vi "CAN_MotorControl.vi"(5 "sbCANopenBaseClass in":refnum<class "sbCANopenBaseClass.lvclass">, 6 "Current":i32=10, 7 "error in (no error)":errorcluster) -> (0 "CANopen Session Out":refnum<class "sbCANopenBaseClass.lvclass">, 1 "Status":T2, 2 "Data Output":T1, 3 "Actual Velocity":i32, 4 "error out":errorcluster)   [LabVIEW 2017]
uses:
  <vilib>/addons/Maxon Motor/EPOS2 CANopen/CANopen/sbCANopenBaseClass.lvclass
  <vilib>/addons/Maxon Motor/EPOS2 CANopen/EPOS2 Support Files/Typedefs/EPOS2 Status Word PVM.ctl
  <vilib>/addons/Maxon Motor/EPOS2 CANopen/EPOS2 Support Files/Typedefs/EPOS2 Data Output Current.ctl
  <vilib>/addons/Maxon Motor/EPOS2 CANopen/EPOS2 Support Files/Typedefs/EPOS2 Control Word PVM.ctl
  <vilib>/addons/Maxon Motor/EPOS2 CANopen/EPOS2 Support Files/Polymorphic SubVIs/Write PDO/EPOS2 Current Mode Write.vi
  <vilib>/addons/Maxon Motor/EPOS2 CANopen/EPOS2 Support Files/Polymorphic SubVIs/Read PDO/EPOS2 Current Mode Read.vi
  <vilib>/addons/Maxon Motor/EPOS2 CANopen/EPOS2 Library.lvlib
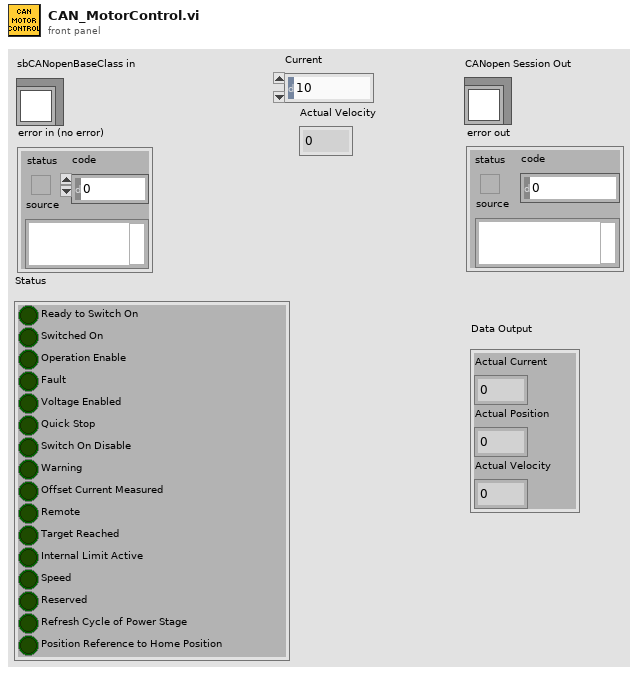
[diagram p1: front panel]
types:
  T1 = typedef "EPOS2 Library.lvlib/EPOS2 Data Output Current.ctl" = cluster{"Actual Current":i16, "Actual Position":i32, "Actual Velocity":i32}
  T2 = typedef "EPOS2 Library.lvlib/EPOS2 Status Word PVM.ctl" = cluster{"Ready to Switch On":bool, "Switched On":bool, "Operation Enable":bool, "Fault":bool, "Voltage Enabled":bool, "Quick Stop":bool, "Switch On Disable":bool, "Warning":bool, "Offset Current Measured":bool, "Remote":bool, "Target Reached":bool, "Internal Limit Active":bool, "Speed":bool, "Reserved":bool, "Refresh Cycle of Power Stage":bool, "Position Reference to Home Position":bool}
  T3 = typedef "EPOS2 Library.lvlib/EPOS2 Control Word PVM.ctl" = cluster{"Switch On":bool, "Enable Voltage":bool, "Quick Stop":bool, "Enable Operation":bool, "Reserved 0":bool, "Reserved 1":bool, "Reserved 2":bool, "Fault Reset":bool, "Halt":bool}
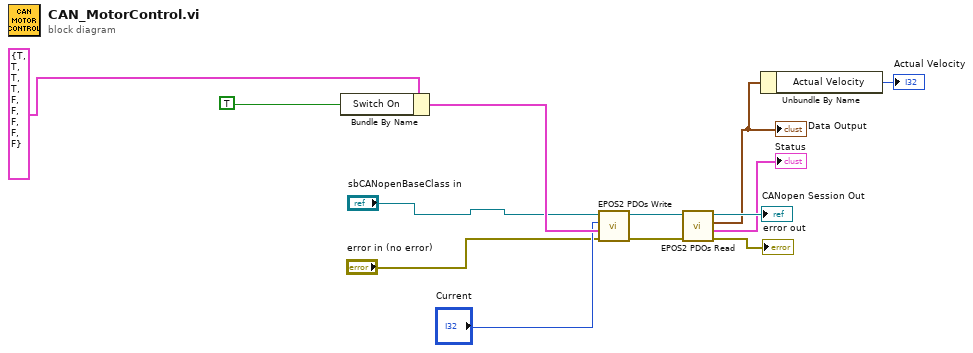
[diagram p0: block diagram]
diagram:
  n1 = Bundle By Name(cluster=T3 {"Switch On"=TRUE, "Enable Voltage"=TRUE, "Quick Stop"=TRUE, "Enable Operation"=TRUE, "Reserved 0"=FALSE, "Reserved 1"=FALSE, "Reserved 2"=FALSE, "Fault Reset"=FALSE, "Halt"=FALSE} ("Control Word"), "Switch On"=TRUE) -> (w12:T3)
  n2 = call-poly <vilib>:"EPOS2 PDOs Write.vi"("error in"="error in (no error)", "Control Word"=w12, "Current"="Current", "CANopen Session In"="sbCANopenBaseClass in") -> ("error out"=w9:errorcluster, "CANopen Session Out"=w11:refnum<class "sbCANopenBaseClass.lvclass">)  [unwired: 6 in]
  n3 = call-poly <vilib>:"EPOS2 PDOs Read.vi"("error in"=w9, "CANopen Session In"=w11) -> ("error out"=→"error out":errorcluster, "Statusword"=→"Status":T2, "Data Output"=w4:T1, "CANopen Session Out"=→"CANopen Session Out":refnum<class "sbCANopenBaseClass.lvclass">)  [unwired: 6 in]
  "Data Output" <- w4
  n4 = Unbundle By Name(w4) -> ("Actual Velocity"=→"Actual Velocity":i32)
